vi "按键捕捉实验.vi"() -> ()   [LabVIEW 2011]
uses:
  <vilib>/eio/EIO_TerminalDirection.ctl
  <vilib>/STM32_DriverVI_Interface_F4/GPIO_EIO/GPI_EIO_Inner_F4.vi
  <vilib>/eio/EIONode/EIONode.xnode
panel:
  out "KEYDOWN":dbl
  in  "停止":bool
  out "数值":i32
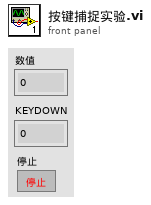
[diagram p1: front panel]
types:
  T1 = enum8{"P0", "P1", "P2", "P3", "P4", "P5", "P6", "P7", "P8", "P9", "P10", "P11", "P12", "P13", "P14", "P15"}
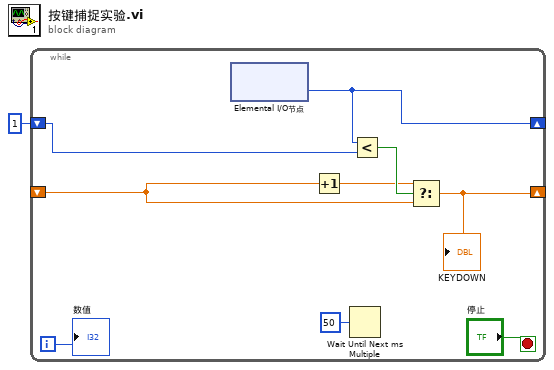
[diagram p0: block diagram]
diagram:
  n1 = while {
    shift-right: [w7] -> _
    shift-left: u8 1 ("KEY_1") -> [w8]
    shift-right: [w4] -> _
    shift-left: _ -> [w2]
    i -> [w10]
    stop <- "停止" stop-if-true
    n2 = xnode "Elemental I/O节点"() -> ("KEY_1"=w7:u8)  [unwired: 1 in, 1 out]
    n3 = Increment(x=w2) -> (x+1=w3:dbl)
    n4 = Wait Until Next ms Multiple(millisecond multiple=u32 50 ("毫秒倍数")) -> ()  [unwired: 1 out]
    n5 = Less?(x=w7, y=w8) -> (x < y?=w5:bool)
    n6 = Select(t=w3, s=w5, f=w2) -> (s? t:f=w4:dbl)
    "KEYDOWN" <- w4
    "数值" <- w10
  }
